vi "Read Initial Frequency and Phase.vi"(8 "error in (no error)":errorcluster, 11 "SV Function in":refnum<class "SV Function.lvclass">) -> (0 "error out":errorcluster, 1 "initial phase":dbl, 2 "initial frequency":dbl, 3 "SV Function out":refnum<class "SV Function.lvclass">, 4 "found?":bool)   [LabVIEW 2017, in "SV Function.lvclass"]
uses:
  <vilib>/addons/_NISVFA/_Generation/Signal Generation/SV Function/SV Function.lvclass
  <vilib>/addons/_NISVFA/_Generation/Signal Generation/SV Function/SV Function.lvclass/SV Function.ctl
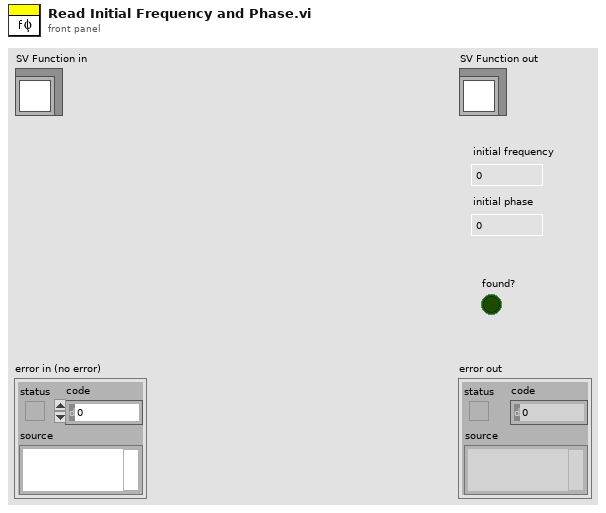
[diagram p1: front panel]
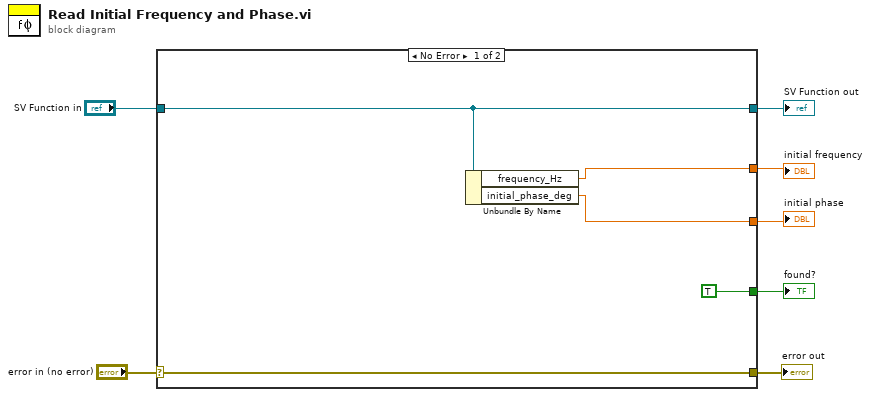
[diagram p0: block diagram]
diagram:
  n1 = case shown="No Error" "error in (no error)" {
    selector: "error in (no error)" -> [w12 w14]
    tunnel: [w12 w14] -> w4
    tunnel: [w10 w13] -> w1
    tunnel: "SV Function in" -> [w10 w13]
    tunnel: [TRUE ("found?") _] -> w5
    tunnel: [w9 _] -> w3
    tunnel: [w8 _] -> w2
    frame No Error {
      n2 = Unbundle By Name(w10) -> ("frequency_Hz"=w8:dbl, "initial_phase_deg"=w9:dbl)
    }
    frame Error {
    }
  }
  "error out" <- w4
  "SV Function out" <- w1
  "initial frequency" <- w2
  "initial phase" <- w3
  "found?" <- w5
